vi "Set Constants Default.vi"(8 "error in (no error)":errorcluster, 10 "Constants":T1={"Port Layout"={"RightMotorInverted"=FALSE, "LeftMotorInverted"=FALSE, "Left Motors"=enum."PWM 0", "Right Motors"=enum."PWM 0", "Auton List"=[], "XBOX Port"=enum."USB 0", "Encoder L A"=enum."DIO 0", "Encoder L B"=enum."DIO 0", "Encoder R A"=enum."DIO 0", "Encoder R B"=enum."DIO 0", "L Encoder Inverse"=FALSE, "R Encoder Inverse"=FALSE, "Drive Distance per Count"=0.0, "Gyro Bus"=enum."SPI On-Board, CS0", "Fuel Roller 1"=enum."PWM 0", "Front Roller"=enum."PWM 0", "Gear Flipper"=enum."PWM 0", "Climber 1"=enum."PWM 0", "Fuel Roller Invert"=FALSE, "Front Roller Invert"=FALSE, "Gear Flipper Invert"=FALSE, "Climber Invert"=FALSE, "PCM"=0, "Fuel Roller 2"=enum."PWM 0", "Gear Sensor"=enum."AI 0", "Gear Release Fwd"=enum."Solenoid 0", "Gear Release Rvrs"=enum."Solenoid 0", "Fuel Arm Fwd"=enum."Solenoid 0", "Fuel Arm Rvrs"=enum."Solenoid 0", "Shifter Fwrd"=enum."Solenoid 0", "Shifter Rvrs"=enum."Solenoid 0", "Climber 2"=enum."PWM 0", "PDP"=60, "Shooter Front Channel"=0, "Shooter Rear Channel"=0, "Shooter Feed Channel"=0, "Camera Servo"=enum."PWM 0", "Gear Servo"=enum."PWM 0", "Gear Puncher Fwrd"=enum."Solenoid 0", "Gear Puncher Rvrs"=enum."Solenoid 0", "Shooter Inverse"=TRUE, "Ring Light Switch"=enum."DIO 4"}, "Drive Constants"={"Wheelbase In."=0.0, "Max Velocity (In/sec)"=0.0, "Max Accel (In/sec^2)"=78.0, "Max Jerk (In/sec^3)"=0.0, "Path dt"=0.0, "Path Sample Count"=0, "Deadband"=0.35}, "Arm System"={"Front Roller Gear Speed"=0.0, "Front Roller Fuel Speed"=0.0, "Gear Flipper Speed"=0.0, "Fuel Roller Speed"=0.0, "Gear Release Wait (ms)"=0, "Gear Sensor Threshold"=0.0, "Flappy Open Angle"=0, "Flappy Close Angle"=0, "Ramp Rate (EGU/min)"=200.0}, "Shooter"={"Shooter Wheels"={"P"=0.0, "I"=0.0, "D"=0.0, "F"=0.0, "IZone"=0.0}, "Feeder"={"P"=0.0, "I"=0.0, "D"=0.0, "F"=0.0, "IZone"=0.0}, "Front Shooter RPM"=0.0, "Rear Shooter RPM"=0.0, "Agitator Speed"=0.0, "Feeder Speed"=0.0, "Shooter CPR"=0, "Feeder CPR"=0}, "Vision"={"High Goal Height (in.)"=0.0, "Low Goal Height (in.)"=0.0, "Camera Height High (in.)"=0.0, "Camera Height Low (in.)"=0.0, "Servo Pitch Gear (deg)"=0.0, "Camera Yaw (deg)"=0.0, "Servo Gear"=0, "Servo Boiler"=0, "Servo Pitch Boiler (deg)"=0.0}}, 11 "selected path":path) -> (0 "error out":errorcluster)   [LabVIEW 2016]
uses:
  Constants/Typedef/Constants.ctl
  <vilib>/Rock Robotics/SystemInterfaces/DIO/FPGA_DIOPWMChannel.ctl
  <vilib>/Rock Robotics/WPI/Joystick/WPI_JoystickDeviceEnum.ctl
  <vilib>/Rock Robotics/SystemInterfaces/DIO/FPGA_DIOChannel.ctl
  <vilib>/Rock Robotics/SystemInterfaces/spilib/spi_bus.ctl
  <vilib>/Rock Robotics/SystemInterfaces/AI/FPGA_AIChannel.ctl
  <vilib>/Rock Robotics/WPI/Solenoid/WPI_SolenoidChannel.ctl
  Constants/Constants.lvlib
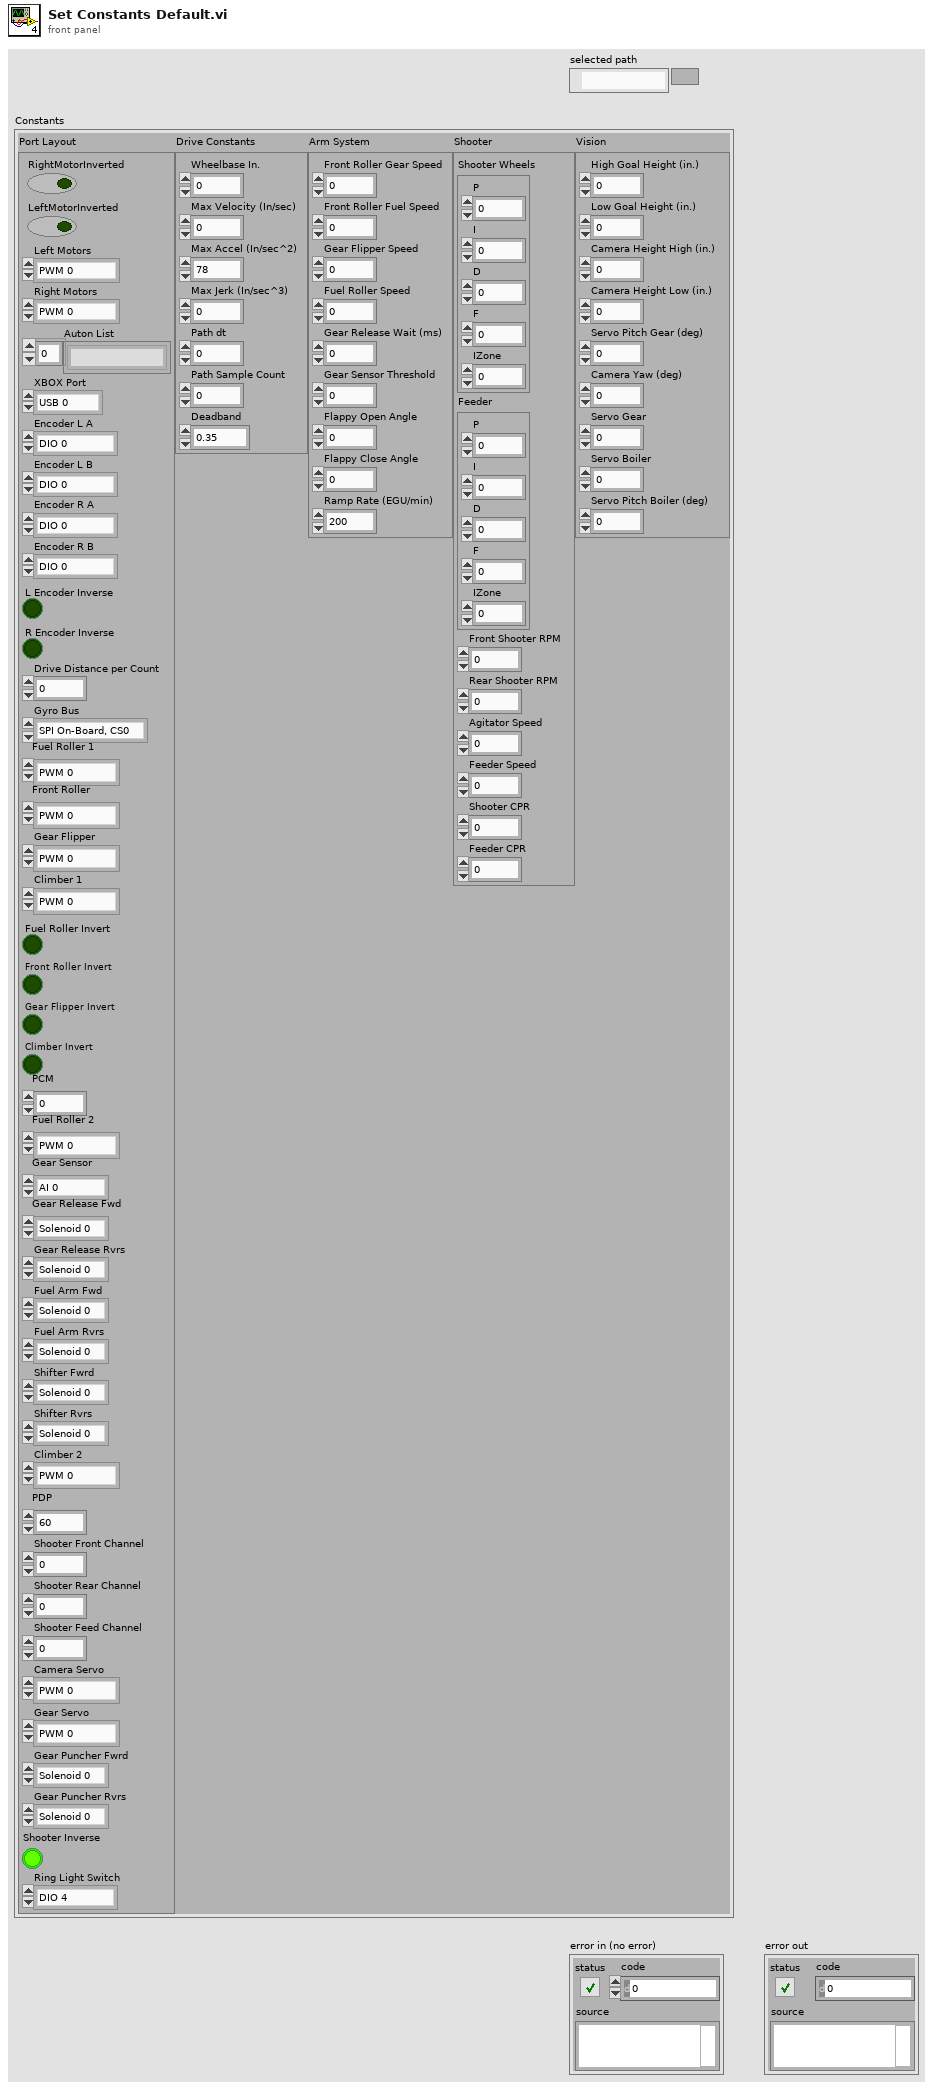
[diagram p1: front panel]
types:
  T1 = typedef "Constants.lvlib/Constants.ctl" = cluster{"Port Layout":cluster{"RightMotorInverted":bool, "LeftMotorInverted":bool, "Left Motors":T2, "Right Motors":T2, "Auton List":string[], "XBOX Port":T3, "Encoder L A":T4, "Encoder L B":T4, "Encoder R A":T4, "Encoder R B":T4, "L Encoder Inverse":bool, "R Encoder Inverse":bool, "Drive Distance per Count":dbl, "Gyro Bus":T5, "Fuel Roller 1":T2, "Front Roller":T2, "Gear Flipper":T2, "Climber 1":T2, "Fuel Roller Invert":bool, "Front Roller Invert":bool, "Gear Flipper Invert":bool, "Climber Invert":bool, "PCM":u8, "Fuel Roller 2":T2, "Gear Sensor":T6, "Gear Release Fwd":T7, "Gear Release Rvrs":T7, "Fuel Arm Fwd":T7, "Fuel Arm Rvrs":T7, "Shifter Fwrd":T7, "Shifter Rvrs":T7, "Climber 2":T2, "PDP":u8, "Shooter Front Channel":u8, "Shooter Rear Channel":u8, "Shooter Feed Channel":u8, "Camera Servo":T2, "Gear Servo":T2, "Gear Puncher Fwrd":T7, "Gear Puncher Rvrs":T7, "Shooter Inverse":bool, "Ring Light Switch":T4}, "Drive Constants":cluster{"Wheelbase In.":dbl, "Max Velocity (In/sec)":dbl, "Max Accel (In/sec^2)":dbl, "Max Jerk (In/sec^3)":dbl, "Path dt":dbl, "Path Sample Count":i32, "Deadband":dbl}, "Arm System":cluster{"Front Roller Gear Speed":dbl, "Front Roller Fuel Speed":dbl, "Gear Flipper Speed":dbl, "Fuel Roller Speed":dbl, "Gear Release Wait (ms)":i32, "Gear Sensor Threshold":dbl, "Flappy Open Angle":i32, "Flappy Close Angle":i32, "Ramp Rate (EGU/min)":dbl}, "Shooter":cluster{"Shooter Wheels":cluster{"P":dbl, "I":dbl, "D":dbl, "F":dbl, "IZone":dbl}, "Feeder":cluster{"P":dbl, "I":dbl, "D":dbl, "F":dbl, "IZone":dbl}, "Front Shooter RPM":dbl, "Rear Shooter RPM":dbl, "Agitator Speed":dbl, "Feeder Speed":dbl, "Shooter CPR":u32, "Feeder CPR":u32}, "Vision":cluster{"High Goal Height (in.)":dbl, "Low Goal Height (in.)":dbl, "Camera Height High (in.)":dbl, "Camera Height Low (in.)":dbl, "Servo Pitch Gear (deg)":dbl, "Camera Yaw (deg)":dbl, "Servo Gear":i32, "Servo Boiler":i32, "Servo Pitch Boiler (deg)":dbl}}
  T2 = typedef "FPGA_DIOPWMChannel.ctl" = enum8{"PWM 0", "PWM 1", "PWM 2", "PWM 3", "PWM 4", "PWM 5", "PWM 6", "PWM 7", "PWM 8", "PWM 9", "PWM MXP 0", "PWM MXP 1", "PWM MXP 2", "PWM MXP 3", "PWM MXP 4", "PWM MXP 5", "PWM MXP 6", "PWM MXP 7", "PWM MXP 8", "PWM MXP 9", "Invalid"}
  T3 = typedef "WPI_JoystickDeviceEnum.ctl" = enum16{"USB 0", "USB 1", "USB 2", "USB 3", "USB 4", "USB 5"}
  T4 = typedef "FPGA_DIOChannel.ctl" = enum8{"DIO 0", "DIO 1", "DIO 2", "DIO 3", "DIO 4", "DIO 5", "DIO 6", "DIO 7", "DIO 8", "DIO 9", "DIO MXP 0", "DIO MXP 1", "DIO MXP 2", "DIO MXP 3", "DIO MXP 4", "DIO MXP 5", "DIO MXP 6", "DIO MXP 7", "DIO MXP 8", "DIO MXP 9", "DIO MXP 10", "DIO MXP 11", "DIO MXP 12", "DIO MXP 13", "DIO MXP 14", "DIO MXP 15", "SPI Port CS1", "SPI Port CS2", "SPI Port CS3", "SPI Port MISO", "SPI Port MOSI", "Invalid"}
  T5 = typedef "spi_bus.ctl" = enum16{"SPI On-Board, CS0", "SPI On-Board, CS1", "SPI On-Board, CS2", "SPI On-Board, CS3", "SPI MXP", "Invalid"}
  T6 = typedef "FPGA_AIChannel.ctl" = enum8{"AI 0", "AI 1", "AI 2", "AI 3", "AI MXP 0", "AI MXP 1", "AI MXP 2", "AI MXP 3", "Invalid"}
  T7 = typedef "WPI_SolenoidChannel.ctl" = enum8{"Solenoid 0", "Solenoid 1", "Solenoid 2", "Solenoid 3", "Solenoid 4", "Solenoid 5", "Solenoid 6", "Solenoid 7", "Invalid"}
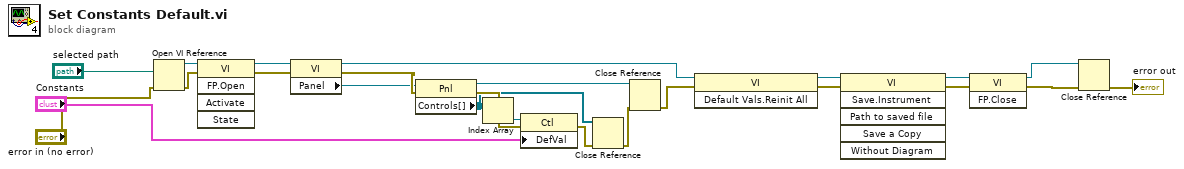
[diagram p0: block diagram]
diagram:
  n1 = Open VI Reference(vi path="selected path", error in (no error)="error in (no error)") -> (vi reference=w11:refnum<vi>, error out=w10:errorcluster)  [unwired: 4 in]
  n2 = invoke class="VI" method="FP.Open"(reference=w11, error in=w10) -> (reference out=w8:refnum<vi>, error out=w9:errorcluster)  [unwired: 3 in, 3 out]
  n3 = property class="VI"(reference=w8, error in=w9) -> (reference out=w4:refnum<vi>, error out=w22:errorcluster, "Panel"=w12:refnum<vi>)
  n4 = property class="Pnl"(reference=w12, error in=w22) -> (reference out=w15:refnum<vi>, error out=w21:errorcluster, "Controls[]"=w16:refnum<vi>[])
  n5 = Index Array(array=w16) -> (element=w14:refnum<vi>)  [unwired: 1 in]
  n6 = property class="Ctl"(reference=w14, error in=w21, "DefVal"="Constants") -> (error out=w17:errorcluster)  [unwired: 1 out]
  n7 = Close Reference(reference=w16, error in (no error)=w17) -> (error out=w18:errorcluster)
  n8 = Close Reference(reference=w15, error in (no error)=w18) -> (error out=w19:errorcluster)
  n9 = invoke class="VI" method="Default Vals.Reinit All"(reference=w4, error in=w19) -> (reference out=w2:refnum<vi>, error out=w5:errorcluster)  [unwired: 1 in, 1 out]
  n10 = invoke class="VI" method="Save.Instrument"(reference=w2, error in=w5) -> (reference out=w1:refnum<vi>, error out=w3:errorcluster)  [unwired: 4 in, 4 out]
  n11 = invoke class="VI" method="FP.Close"(reference=w1, error in=w3) -> (reference out=w6:refnum<vi>, error out=w7:errorcluster)  [unwired: 1 in, 1 out]
  n12 = Close Reference(reference=w6, error in (no error)=w7) -> (error out=→"error out":errorcluster)
